vi "Dequeue Results.vi"(11 "Result Model by Reference in":refnum<class "Result Model by Reference.lvclass">) -> (3 "Result Model by Reference out":refnum<class "Result Model by Reference.lvclass">)   [LabVIEW 2020, in "Result Model by Reference.lvclass"]
uses:
  Result Model by Reference.lvclass
  Result Model by Reference.lvclass/Result Model by Reference.ctl
  Result Model/Result Model.lvclass
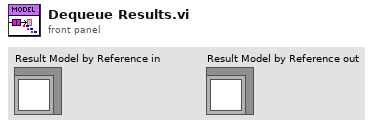
[diagram p1: front panel]
types:
  T1 = typedef "Result.lvlib/Result.ctl" = cluster{"Name":string, "Message":string, "Description":string, "Status":T2, "Result Type":T3, "Execution Time":dbl}
  T2 = typedef "Result.lvlib/Status.ctl" = enum16{"", "Passed", "Failed", "Error", "Skipped", "Setup Error", "Broken", "Teardown Error"}
  T3 = typedef "Result.lvlib/Type.ctl" = enum16{"Test Case", "Test Suite", "Test Run", "Pass", "Fail", "Skip", "Pass if", "Fail if", "Pass if Error", "Fail if Error", "Pass if Equal", "Fail if Equal"}
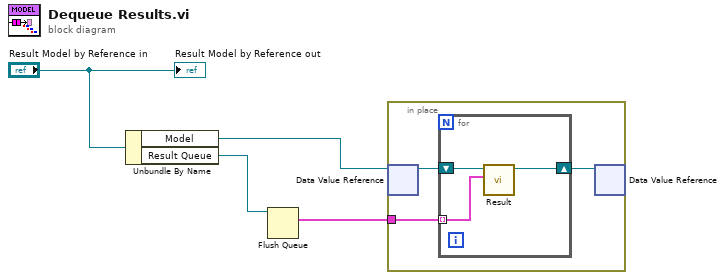
[diagram p0: block diagram]
diagram:
  n1 = Unbundle By Name("Result Model by Reference in") -> ("Model"=w4:refnum<data-value>, "Result Queue"=w2:refnum<queue>)
  n2 = Flush Queue(queue=w2) -> (remaining elements=w1:T1[])  [unwired: 1 in, 2 out]
  n3 = in-place {
    in-place-border: w1 -> [w5]
    n4 = in-place-dvr #1(w4) -> (w6:refnum<class "Result Model.lvclass">)  [unwired: 1 out]
    n5 = for {
      shift-right: [w10] -> w7
      shift-left: w6 -> [w9]
      tunnel: w5 -> [w8] mode=indexing
      n6 = call-dynamic "Result.vi"("Results"=w8, "Result Model In"=w9) -> ("Result Model Out"=w10:refnum<class "Result Model.lvclass">)  [unwired: 8 in, 1 out]
    }
    n7 = in-place-dvr #1(w7) -> ()  [unwired: 2 out]
  }
  "Result Model by Reference out" <- "Result Model by Reference in"
